vi "FT10_Log Queue Data.vi"(11 "Message Handling Cluster in":T1) -> (3 "Message Handling Cluster out":T1)   [LabVIEW 2015]
uses:
  Controls/Control_Message Handling Cluster.ctl
  Controls/Control_M4X Connection.ctl
  Controls/Control_PXI-7854R FPGA Reference.ctl
  Controls/Control_Config Cluster.ctl
  Controls/Control_Config Unitherm Port.ctl
  Controls/Control_Config Simulate Values.ctl
  Controls/Control_Log Queue.ctl
  Controls/Control_Log Cluster.ctl
  Controls/Control_Log Time.ctl
  Controls/Control_Log Waveform Cluster.ctl
  Controls/Control_Log Analysis Cluster.ctl
  Controls/Control_Log Flag.ctl
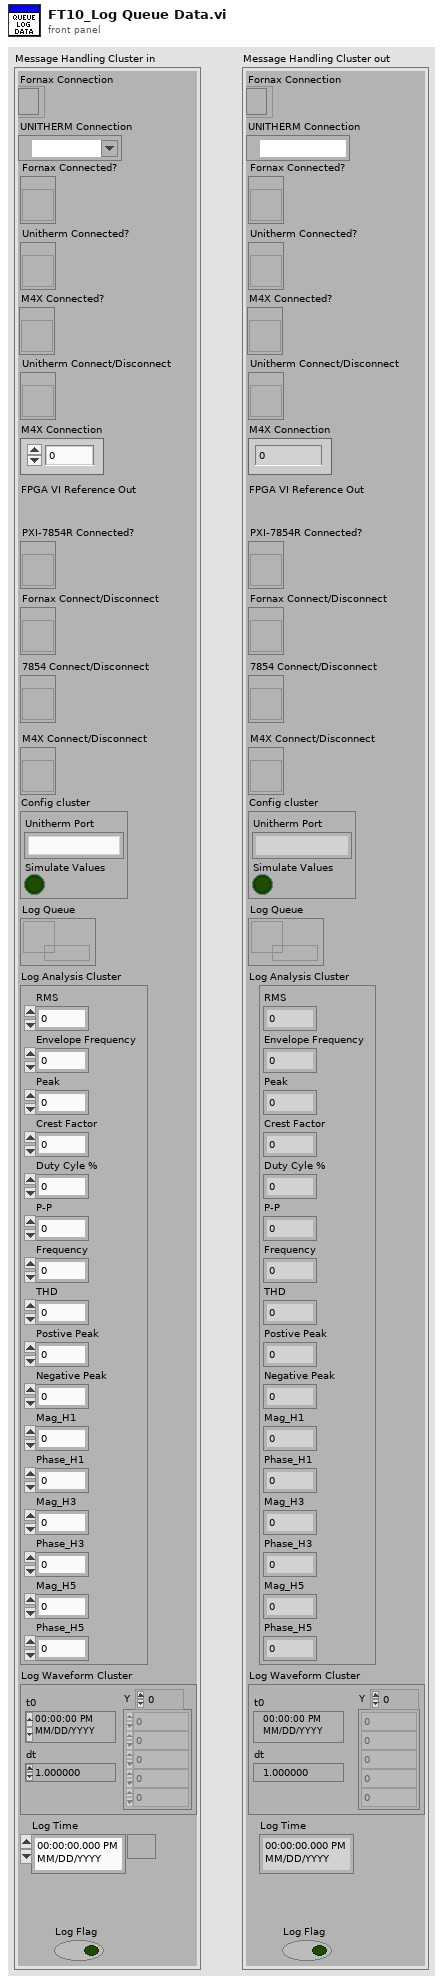
[diagram p1: front panel]
types:
  T1 = typedef "Control_Message Handling Cluster.ctl" = cluster{"Fornax Connected?":refnum<vi>, "Unitherm Connected?":refnum<vi>, "M4X Connected?":refnum<vi>, "Unitherm Connect/Disconnect":refnum<vi>, "Fornax Connection":refnum<k5>, "UNITHERM Connection":refnum<visa-resource-name>, "M4X Connection":T2, "PXI-7854R FPGA Reference":T3, "PXI-7854R Connected?":refnum<vi>, "Fornax Connect/Disconnect":refnum<vi>, "7854 Connect/Disconnect":refnum<vi>, "M4X Connect/Disconnect":refnum<vi>, "Config Cluster":T4, "Log Queue":T7, "Log Analysis Cluster":T8, "Log Waveform Cluster":T9, "Log Time":T10, "Log Flag":T11}
  T2 = typedef "Control_M4X Connection.ctl" = u32
  T3 = typedef "Control_PXI-7854R FPGA Reference.ctl" = refnum<k20>
  T4 = typedef "Control_Config Cluster.ctl" = cluster{"Unitherm Port":T5, "Simulate Values":T6}
  T5 = typedef "Control_Config Unitherm Port.ctl" = string
  T6 = typedef "Control_Config Simulate Values.ctl" = bool
  T7 = typedef "Control_Log Queue.ctl" = refnum<queue>
  T8 = typedef "Control_Log Analysis Cluster.ctl" = cluster{"RMS":dbl, "Envelope Frequency":dbl, "Peak":dbl, "Crest Factor":dbl, "Duty Cyle %":dbl, "P-P":dbl, "Frequency":dbl, "THD":dbl, "Postive Peak":dbl, "Negative Peak":dbl, "Mag_H1":dbl, "Phase_H1":dbl, "Mag_H3":dbl, "Phase_H3":dbl, "Mag_H5":dbl, "Phase_H5":dbl}
  T9 = typedef "Control_Log Waveform Cluster.ctl" = waveform(dbl)
  T10 = typedef "Control_Log Time.ctl" = timestamp
  T11 = typedef "Control_Log Flag.ctl" = bool
  T12 = typedef "Control_Log Cluster.ctl" = cluster{"Log Time":T10, "Log Waveform Cluster":T9, "Log Analysis Cluster":T8}
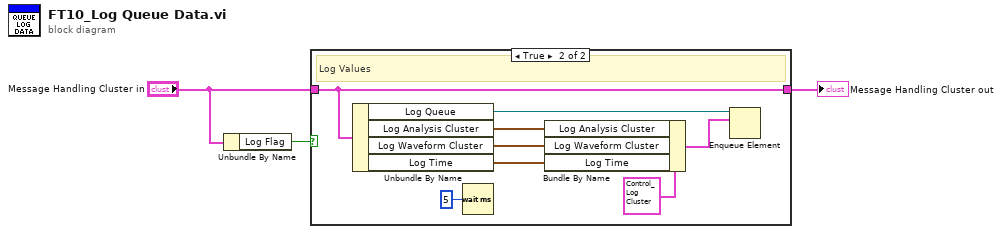
[diagram p0: block diagram]
diagram:
  n1 = Unbundle By Name("Message Handling Cluster in") -> ("Log Flag"=w3:T11)
  n2 = case shown="True" w3 {
    tunnel: "Message Handling Cluster in" -> [w4 w11]
    tunnel: [w4 w11] -> w1
    frame False {
      # "Do nothing"
    }
    frame True {
      # "Log Values"
      n3 = Unbundle By Name(w11) -> ("Log Queue"=w12:T7, "Log Analysis Cluster"=w9:T8, "Log Waveform Cluster"=w8:T9, "Log Time"=w7:T10)
      n4 = Wait (ms)(milliseconds to wait=u32 5) -> ()  [unwired: 1 out]
      n5 = Bundle By Name(cluster=T12 {"Log Time"=timestamp(0 s since 1904-01-01), "Log Waveform Cluster"={"t0"=timestamp(0 s since 1904-01-01), "dt"=1.0, "Y"=[]}, "Log Analysis Cluster"={"RMS"=0.0, "Envelope Frequency"=0.0, "Peak"=0.0, "Crest Factor"=0.0, "Duty Cyle %"=0.0, "P-P"=0.0, "Frequency"=0.0, "THD"=0.0, "Postive Peak"=0.0, "Negative Peak"=0.0, "Mag_H1"=0.0, "Phase_H1"=0.0, "Mag_H3"=0.0, "Phase_H3"=0.0, "Mag_H5"=0.0, "Phase_H5"=0.0}} ("Cluster"), "Log Analysis Cluster"=w9, "Log Waveform Cluster"=w8, "Log Time"=w7) -> (w6:T12)
      n6 = Enqueue Element(queue=w12, element=w6) -> ()  [unwired: 2 in, 3 out]
    }
  }
  "Message Handling Cluster out" <- w1
